vi "Simple Test.vi"() -> ()   [LabVIEW 2016]
panel:
  out "x+1":dbl
  in  "Numeric":dbl
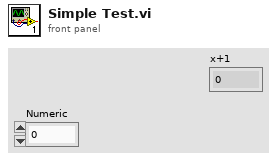
[diagram p1: front panel]
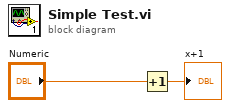
[diagram p0: block diagram]
diagram:
  n1 = Increment(x="Numeric") -> (x+1=→"x+1":dbl)
